vi "Group_SetupTDMS.vi"(8 "error in (no error)":errorcluster, 10 "tdms file in":refnum<k34>, 11 "Group in":refnum<class "Group.lvclass">) -> (0 "error out":errorcluster, 2 "tdms file out":refnum<k34>, 3 "Group out":refnum<class "Group.lvclass">)   [LabVIEW 2023, in "Group.lvclass"]
doc: "Adds the group and group properties to the specified TDMS file."
uses:
  Group.lvclass
  Group.lvclass/Group.ctl
  Channel/Channel.lvclass
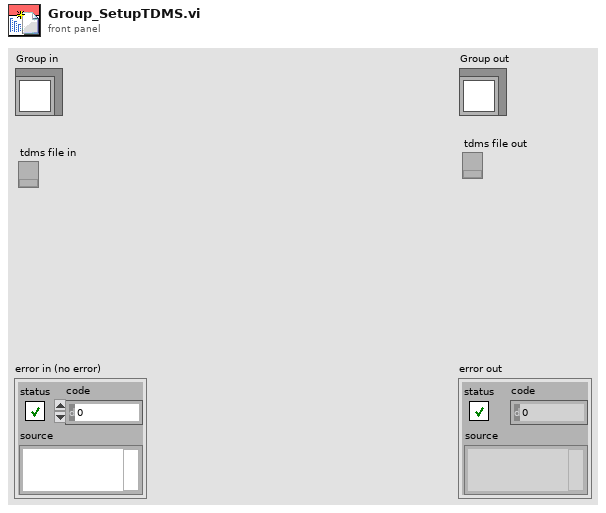
[diagram p1: front panel]
types:
  T1 = typedef "Meta Data.ctl" = cluster{"Key":string, "Value":string}
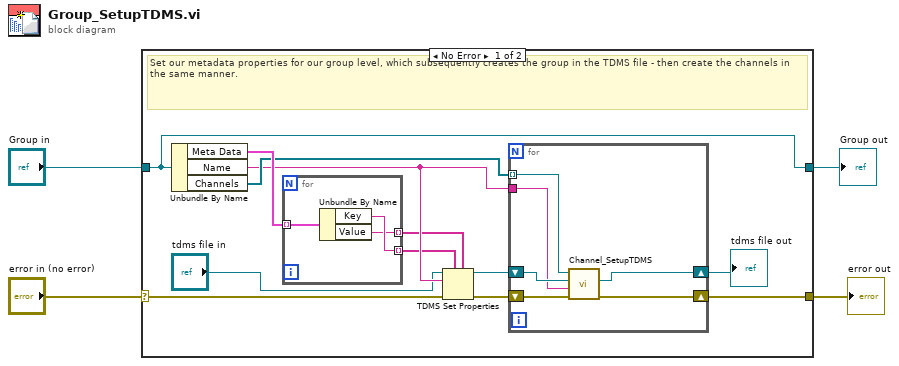
[diagram p0: block diagram]
diagram:
  n1 = case shown="No Error" "error in (no error)" {
    selector: "error in (no error)" -> [w7 w27]
    tunnel: [w12 w27] -> w3
    tunnel: [w16 w26] -> w1
    tunnel: "Group in" -> [w16 w26]
    frame No Error {
      # "Set our metadata properties for our group level, which subsequently creates the group in the TDMS file - then create the channels in the same manner."
      n2 = Unbundle By Name(w16) -> ("Meta Data"=w15:T1[], "Name"=w13:string, "Channels"=w14:refnum<class "Channel.lvclass">[])
      n3 = for {
        tunnel: w15 -> [w25] mode=indexing
        tunnel: [w24] -> w6 mode=indexing
        tunnel: [w23] -> w5 mode=indexing
        n4 = Unbundle By Name(w25) -> ("Key"=w24:string, "Value"=w23:string)
      }
      n5 = TDMS Set Properties(5:w5, 7:w6, 8:w7, 10:w13, 11:"tdms file in") -> (0:w8:errorcluster, 3:w9:refnum<k34>)  [unwired: 1 in, 2 out]
      n6 = for {
        tunnel: w14 -> [w22] mode=indexing
        shift-right: [w18] -> w12
        shift-left: w8 -> [w21]
        tunnel: w13 -> [w19]
        shift-right: [w17] -> w11
        shift-left: w9 -> [w20]
        n7 = call-dynamic "Channel_SetupTDMS.vi"("error in (no error)"=w21, "Group Name"=w19, "tdms file in"=w20, "Channel in"=w22) -> ("error out"=w18:errorcluster, "tdms file out"=w17:refnum<k34>)  [unwired: 5 in, 1 out]
      }
      "tdms file out" <- w11
    }
    frame Error {
    }
  }
  "error out" <- w3
  "Group out" <- w1
